vi "stopMotion.vi"(8 "error in (no error)":errorcluster, 11 "Model in":refnum<class "Model.lvclass">) -> (0 "error out":errorcluster, 3 "Model out":refnum<class "Model.lvclass">)   [LabVIEW 2015]
uses:
  <userlib>/Common/Devices/PressureValve/PressureValve/PressureValve.lvclass
  Model.lvclass
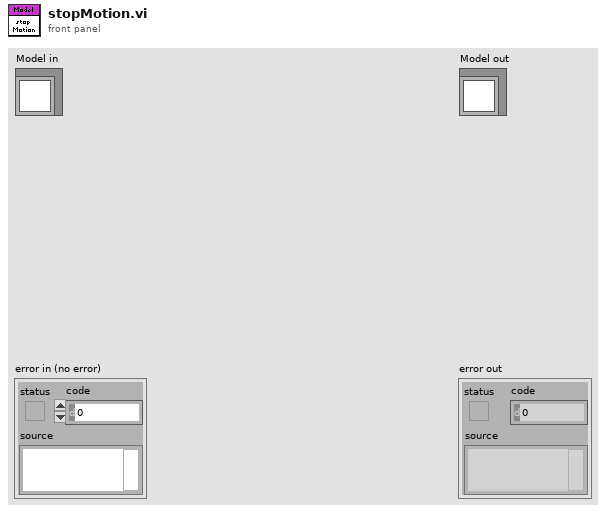
[diagram p1: front panel]
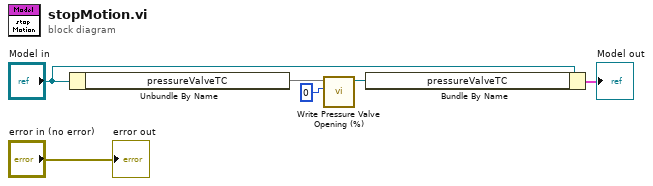
[diagram p0: block diagram]
diagram:
  n1 = Unbundle By Name("Model in") -> ("pressureValveTC"=w3)
  n2 = call <userlib>:"Write Pressure Valve Opening (%).vi"("Pressure Valve Opening (%)"=u16 0 ("Ramp Output"), "PressureValve in"=w3) -> ("PressureValve out"=w2:refnum<class "PressureValve.lvclass">)  [unwired: 9 in]
  n3 = Bundle By Name(cluster="Model in", "pressureValveTC"=w2) -> (→"Model out":cluster{})
  "error out" <- "error in (no error)"
